vi "TestMakeAlotOfLargeArraysAndPutInGraph.vi"() -> ()   [LabVIEW 2017]
panel:
  out "Intensity Graph":dbl[][](graph)
  out "Flip Flop":bool=TRUE
  out "Large Array":dbl[][](array[numeric])
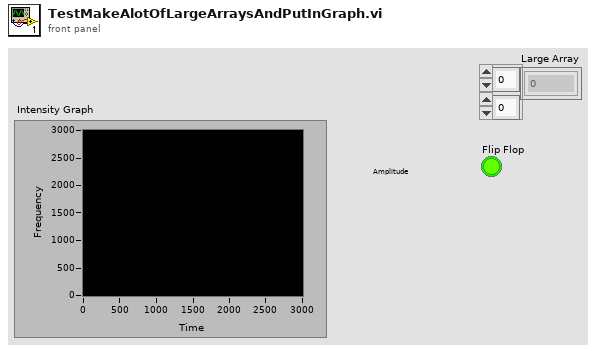
[diagram p1: front panel]
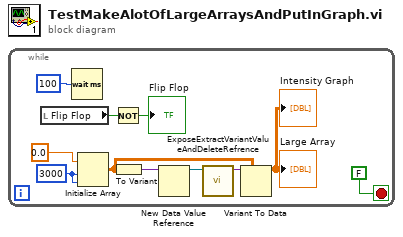
[diagram p0: block diagram]
diagram:
  n1 = while {
    stop <- FALSE stop-if-true
    w8 = 3000 ("dimension size")
    n2 = local read "Flip Flop"() -> (w7:bool)
    n3 = Wait (ms)(milliseconds to wait=u32 100) -> ()  [unwired: 1 out]
    n4 = Initialize Array(0.0 ("element"), w8, w8) -> (w3:dbl[][])
    n5 = Not(x=w7) -> (.not. x?=→"Flip Flop":bool)
    n6 = To Variant(anything=w3) -> (Variant=w5:variant)
    n7 = New Data Value Reference(data value=w5) -> (data value reference=w4:refnum<data-value>)  [unwired: 1 in, 1 out]
    n8 = call "ExposeExtractVariantValueAndDeleteRefrence.vi"("Data Value Reference in"=w4) -> ("Value out"=w2:variant)  [unwired: 10 in]
    n9 = Variant To Data(type=w3, Variant=w2) -> (data=→"Large Array" →"Intensity Graph":dbl[][])  [unwired: 1 in, 1 out]
  }
